vi "Configure Chan Mode (Duty Cycle).vi"(1 "Delay (10 msec)":dbl=0.01 format="%.6p", 2 "Width (10 msec)":dbl=0.01 format="%.6p", 4 "Chan DC Off (10)":i32=10, 6 "Chan DC On (10)":i32=10, 7 "Channel (1:Chan A)":i32(ring)=1 items=["Channel A"=1, "Channel B"=2, "Channel C"=3, "Channel D"=4, "Channel E"=5, "Channel F"=6, "Channel G"=7, "Channel H"=8], 8 "error in (no error)":errorcluster, 9 "Wait # (0)":i32, 11 "VISA resource name":refnum<visa-resource-name>) -> (0 "error out":errorcluster, 3 "VISA resource name out":refnum<visa-resource-name>)   [LabVIEW 2012, in "Berkeley Nucleonics 500 Series.lvlib"]
doc: "This VI is used to configure the duty cycle mode of operation for the selected channel."
uses:
  Berkeley Nucleonics 500 Series.lvlib
  Action-Status/Query Chan Parameters (Mode).vi
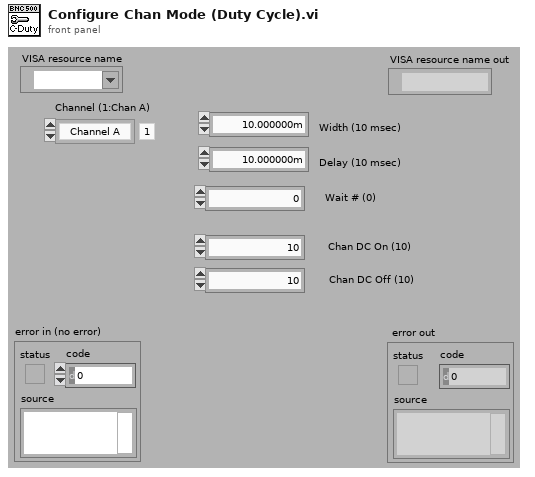
[diagram p1: front panel]
types:
  T1 = enum16{"Normal", "Single", "Burst", "Duty Cycle"}
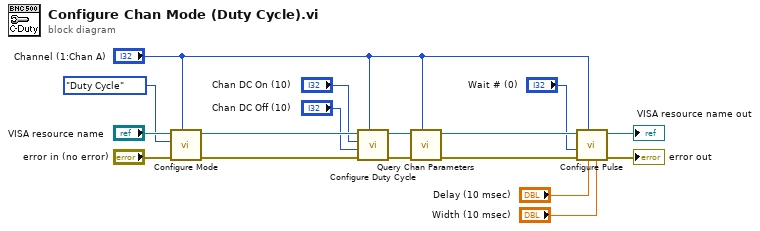
[diagram p0: block diagram]
diagram:
  n1 = call "Configure Mode.vi"("Channel (1:Chan A)"="Channel (1:Chan A)", "error in (no error)"="error in (no error)", "Mode (0:Normal)"=T1."Duty Cycle" ("Chan Mode"), "VISA resource name"="VISA resource name") -> ("error out"=w14:errorcluster, "VISA resource name out"=w15:refnum<visa-resource-name>)  [unwired: 6 out]
  n2 = call "Configure Duty Cycle.vi"("Channel (1:Chan A)"="Channel (1:Chan A)", "error in (no error)"=w14, "DC Off (10)"="Chan DC Off (10)", "DC On (10)"="Chan DC On (10)", "VISA resource name"=w15) -> ("error out"=w10:errorcluster, "VISA resource name out"=w9:refnum<visa-resource-name>)  [unwired: 5 out]
  n3 = call-poly "Query Chan Parameters.vi"("Channel (1: Chan A)"="Channel (1:Chan A)", "error in (no error)"=w10, "VISA resource name"=w9) -> ("error out"=w8:errorcluster, "VISA resource name out"=w7:refnum<visa-resource-name>)  [unwired: 7 out]
  n4 = call "Configure Pulse.vi"("Width (10 msec)"="Width (10 msec)", "Delay (10 msec)"="Delay (10 msec)", "Channel (1:Chan A)"="Channel (1:Chan A)", "error in (no error)"=w8, "Wait # (0)"="Wait # (0)", "VISA resource name"=w7) -> ("error out"=→"error out":errorcluster, "VISA resource name out"=→"VISA resource name out":refnum<visa-resource-name>)  [unwired: 4 out]
